vi "Get Registry Update Event.vi"() -> (2 "Event Registration Refnum":refnum<event-registration>)   [LabVIEW 2020, in "AF Debug.lvlib"]
doc: "This VI returns an Event registration refnum for an Actor Framework debugger to use to hear about changes to the available debug information of actors. Every time this event fires, new information from the database is available for the debugger to harvest and display. The event itself does not carry any information to avoid duplicating information in the Event queue.\n\nThis VI is a wrapper for a VI of the same name in Actor Framework.lvlib. It has been provided to support tools written to use older versions of the AF Debug library. It is DEPRECATED, but functional."
uses:
  AFDebug/AF Debug.lvlib
  Actor Framework.lvlib
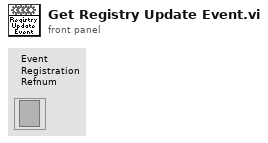
[diagram p1: front panel]
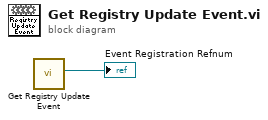
[diagram p0: block diagram]
diagram:
  n1 = call "Get Registry Update Event.vi"() -> ("Event Registration Refnum"=→"Event Registration Refnum":refnum<event-registration>)  [unwired: 11 in]
